vi "vectorizing_text_data.vi"() -> ()   [LabVIEW 2020]
uses:
  <userlib>/_Soliton/LabVIEW LLM Libraries/vectorstore/vector_qdrant/vector_qdrant.lvclass
  C:/Program Files/National Instruments/LabVIEW 2020/user.lib/_Soliton/LabVIEW LLM Libraries/vectorstore/abstract_vector_base/abstract_vector_base.lvclass
  <userlib>/_Soliton/LabVIEW LLM Libraries/data_destination/destination_vectorstore/destination_vectorstore.lvclass
  C:/Program Files/National Instruments/LabVIEW 2020/user.lib/_Soliton/LabVIEW LLM Libraries/data_destination/abstract_datadestination_base/abstract_datadestination_base.lvclass
  <userlib>/_Soliton/LabVIEW LLM Libraries/models/llm_openai_embedding/llm_openai_embedding.lvclass
  C:/Program Files/National Instruments/LabVIEW 2020/user.lib/_Soliton/LabVIEW LLM Libraries/models/abstract_llm_base/abstract_llm_base.lvclass
  <userlib>/_Soliton/LabVIEW LLM Libraries/data_source/datasource_text_file/datasource_text_file.lvclass
  C:/Program Files/National Instruments/LabVIEW 2020/user.lib/_Soliton/LabVIEW LLM Libraries/data_source/abstract_datasource_base/abstract_datasource_base.lvclass
  <userlib>/_Soliton/LabVIEW LLM Libraries/data_processor/chunk_character_splitter/chunk_character_splitter.lvclass
  C:/Program Files/National Instruments/LabVIEW 2020/user.lib/_Soliton/LabVIEW LLM Libraries/data_processor/abstract_dataprocessing_base/abstract_dataprocessing_base.lvclass
  <userlib>/_Soliton/LabVIEW LLM Libraries/data_processor/embed_nodes/embed_nodes.lvclass
  <userlib>/_Soliton/LabVIEW LLM Libraries/models/llm_openai_embedding/Instantiate_llm_openai_embed.vi
  <userlib>/_Soliton/LabVIEW LLM Libraries/data_pipeline/data_simple_pipeline/data_simple_pipeline.lvclass
  <userlib>/_Soliton/LabVIEW LLM Libraries/data_processor/abstract_dataprocessing_base/abstract_dataprocessing_base.lvclass
panel:
  out "error out":errorcluster
  in  "max_character_length":u32=500
  in  "recursive_folder_load":bool=TRUE
  in  "model_name":string(combo)="text-embedding-ada-002"
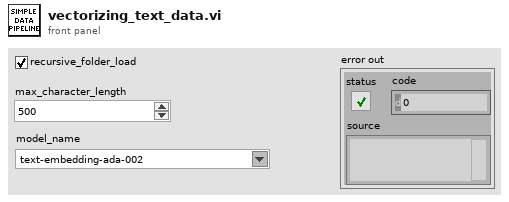
[diagram p1: front panel]
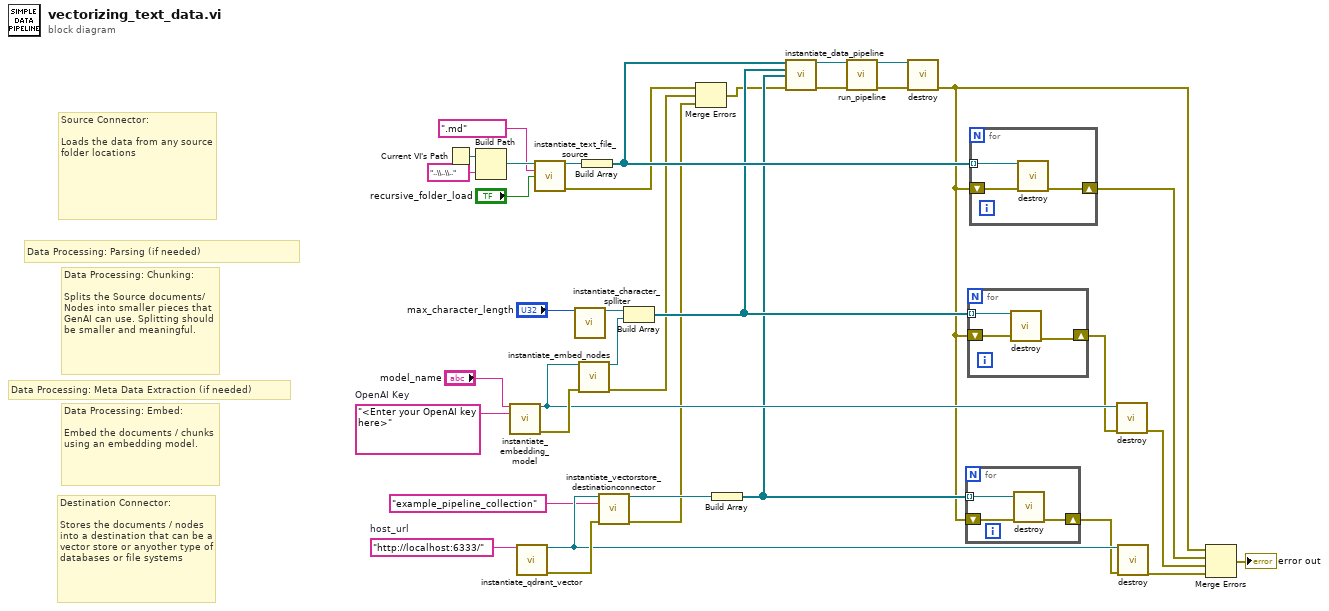
[diagram p0: block diagram]
diagram:
  w24 = "http://localhost:6333/"  # host_url
  w4 = "<Enter your OpenAI key here>"  # OpenAI Key
  # "Destination Connector:\n\nStores the documents / nodes into a destination that can be a vector store or anyother type of databases or file systems"
  # "Data Processing: Meta Data Extraction (if needed)"
  # "Data Processing: Parsing (if needed)"
  # "Data Processing: Embed:\n\nEmbed the documents / chunks using an embedding model."
  # "Data Processing: Chunking:\n\nSplits the Source documents/Nodes into smaller pieces that GenAI can use. Splitting should be smaller and meaningful."
  # "Source Connector:\n\nLoads the data from any source folder locations"
  n1 = Current VI's Path() -> (path=w36:path)
  n2 = Build Path(base path=w36, name or relative path="..\\..\\..") -> (appended path=w34:path)
  n3 = call-poly <userlib>:"instantiate_embedding_model.vi"("model_name"="model_name", "openai_key"=w4) -> ("llm_openai_embedding out"=w29:refnum<class "llm_openai_embedding.lvclass">, "error out"=w30:errorcluster)  [unwired: 12 in]
  n4 = call <userlib>:"instantiate_qdrant_vector.vi"("host_url"=w24) -> ("vector_qdrant out"=w26:refnum<class "vector_qdrant.lvclass">, "error out"=w27:errorcluster)  [unwired: 13 in]
  n5 = call <userlib>:"instantiate_text_file_source.vi"("source_folder"=w34, "file_extension"=".md", "recursive_folder_load"="recursive_folder_load") -> ("datasource_text_file out"=w18:refnum<class "datasource_text_file.lvclass">, "error out"=w16:errorcluster)  [unwired: 11 in]
  n6 = call <userlib>:"instantiate_character_splliter.vi"("max_character_length"="max_character_length") -> ("chunk_character_splitter out"=w15:refnum<class "chunk_character_splitter.lvclass">)  [unwired: 13 in, 1 out]
  n7 = call <userlib>:"instantiate_embed_nodes.vi"("abstract_llm_embedding"=w29, "error in (no error)"=w30) -> ("embed_nodes out"=w14:refnum<class "embed_nodes.lvclass">, "error out"=w2:errorcluster)  [unwired: 12 in]
  n8 = Build Array(w18) -> (w17:refnum<class "datasource_text_file.lvclass">[])
  n9 = call <userlib>:"instantiate_vectorstore_destinationconnector.vi"("abstract_vector_base"=w26, "store_id"="example_pipeline_collection", "error in (no error)"=w27) -> ("destination_vectorstore out"=w11:refnum<class "destination_vectorstore.lvclass">, "error out"=w1:errorcluster)  [unwired: 11 in]
  n10 = Build Array(w15, w14) -> (w13:refnum<class "abstract_dataprocessing_base.lvclass">[])
  n11 = Merge Errors(w16, w2, w1) -> (w3:errorcluster)
  n12 = Build Array(w11) -> (w10:refnum<class "destination_vectorstore.lvclass">[])
  n13 = call <userlib>:"instantiate_data_pipeline.vi"("sources"=w17, "processing steps"=w13, "destinations"=w10, "error in (no error)"=w3) -> ("data_simple_pipeline out"=w22:refnum<class "data_simple_pipeline.lvclass">, "error out"=w21:errorcluster)  [unwired: 10 in]
  n14 = call-dynamic "run_pipeline.vi"("data_simple_pipeline in"=w22, "error in (no error)"=w21) -> ("data_simple_pipeline out"=w20:refnum<class "data_simple_pipeline.lvclass">, "error out"=w19:errorcluster)  [unwired: 12 in]
  n15 = call-dynamic "destroy.vi"("data_simple_pipeline in"=w20, "error in (no error)"=w19) -> ("error out"=w6:errorcluster)  [unwired: 12 in, 1 out]
  n16 = for {
    shift-right: [w39] -> w25
    shift-left: w6 -> [w38]
    tunnel: w10 -> [w37] mode=indexing
    n17 = call-dynamic "destroy.vi"("abstract_datadestination_base in"=w37, "error in (no error)"=w38) -> ("error out"=w39:errorcluster)  [unwired: 12 in, 1 out]
  }
  n18 = for {
    tunnel: w13 -> [w42] mode=indexing
    shift-right: [w40] -> w12
    shift-left: w6 -> [w41]
    n19 = call-dynamic "destroy.vi"("abstract_dataprocessing_base in"=w42, "error in (no error)"=w41) -> ("error out"=w40:errorcluster)  [unwired: 12 in, 1 out]
  }
  n20 = for {
    tunnel: w17 -> [w45] mode=indexing
    shift-right: [w43] -> w7
    shift-left: w6 -> [w44]
    n21 = call-dynamic "destroy.vi"("abstract_datasource_base in"=w45, "error in (no error)"=w44) -> ("error out"=w43:errorcluster)  [unwired: 12 in, 1 out]
  }
  n22 = call-dynamic "destroy.vi"("error in (no error)"=w12, "llm_openai_embedding in"=w29) -> ("error out"=w8:errorcluster)  [unwired: 8 in, 1 out]
  n23 = call-dynamic "destroy.vi"("vector_qdrant in"=w26, "error in (no error)"=w25) -> ("error out"=w9:errorcluster)  [unwired: 12 in, 1 out]
  n24 = Merge Errors(w6, w7, w8, w9) -> (→"error out":errorcluster)
